vi "clean-up-string.vi"(1 "input string":string) -> (0 "string out":string)   [LabVIEW 2016]
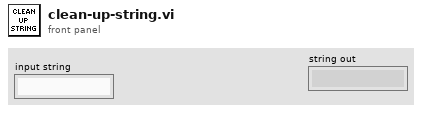
[diagram p1: front panel]
types:
  T1 = enum16{"Native", "Native Command Line", "UNIX", "Macintosh", "DOS"}
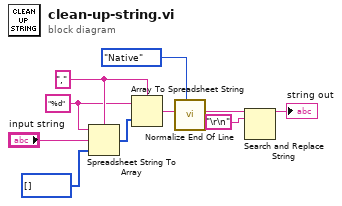
[diagram p0: block diagram]
diagram:
  w6 = "%d" ("format string")
  w7 = "," ("delimiter (Tab)")
  n1 = Spreadsheet String To Array(delimiter (Tab)=w7, format string=w6, spreadsheet string="input string", array type (2D Dbl)=i8[] []) -> (array=w8:i8[])
  n2 = Array To Spreadsheet String(delimiter (Tab)=w7, array=w8, 3:w6) -> (spreadsheet string=w5:string)
  n3 = call <vilib>:"Normalize End Of Line.vi"("end of line (Native)"=T1."Native", "string in"=w5) -> ("string out"=w2:string)  [unwired: 6 in]
  n4 = Search and Replace String(input string=w2, search string="\r\n") -> (result string=→"string out":string)  [unwired: 6 in, 3 out]
